vi "FRCts20_Backend_Test_Event_DELETE.vi"(8 "error in (no error)":errorcluster, 11 "Event Name":string) -> (0 "error out":errorcluster, 1 "Time (ms)":u32, 2 "Status":string, 3 "Event Out":T1, 5 "Success":bool)   [LabVIEW 2013, in "FRCts20_Backend_TestCode.lvlib"]
uses:
  FRCts20_Backend_TestCode.lvlib
  FRCts20_Backend_API/FRCts20_Backend_API_Event.ctl
  FRCts20_Backend_API/FRCts20_Backend_API_SW.ctl
  FRCts20_Backend_API/FRCts20_Backend_API_Command_Event.ctl
  FRCts20_Backend_API/FRCts20_Backend_API_Event.vi
  FRCts20_Backend_API/FRCts20_Backend_API.lvlib
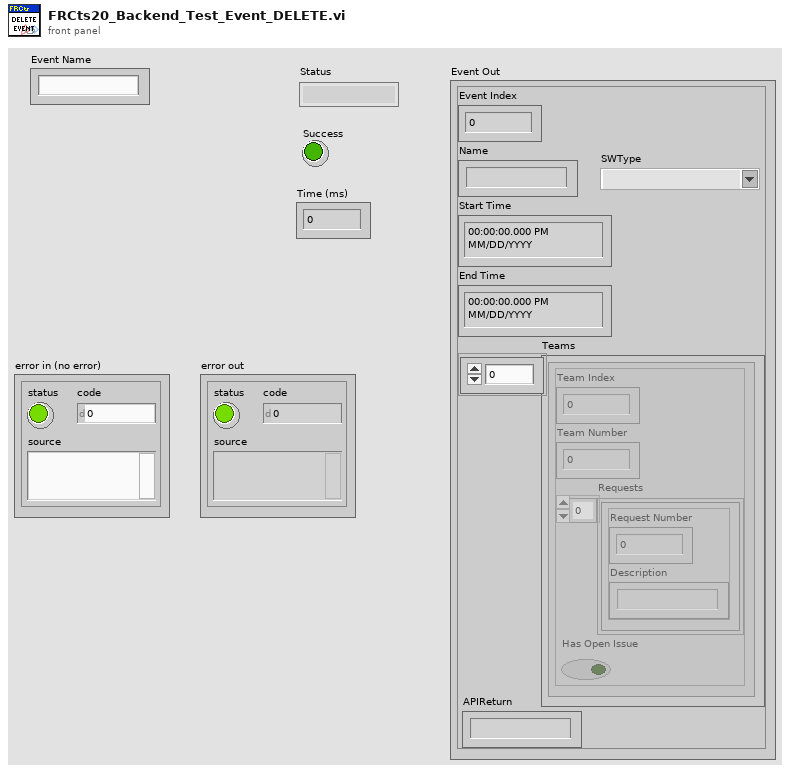
[diagram p1: front panel]
types:
  T1 = typedef "FRCts20_Backend_API.lvlib/FRCts20_Backend_API_Event.ctl" = cluster{"Event Index":u32, "Name":string, "Start Time":timestamp, "End Time":timestamp, "Teams":cluster{"Team Index":u32, "Team Number":u32, "Requests":cluster{"Request Number":u32, "Description":string}[], "Has Open Issue":bool}[], "SWType":T2, "APIReturn":string}
  T2 = typedef "FRCts20_Backend_API.lvlib/FRCts20_Backend_API_SW.ctl" = string
  T3 = typedef "FRCts20_Backend_API.lvlib/FRCts20_Backend_API_Command_Event.ctl" = string
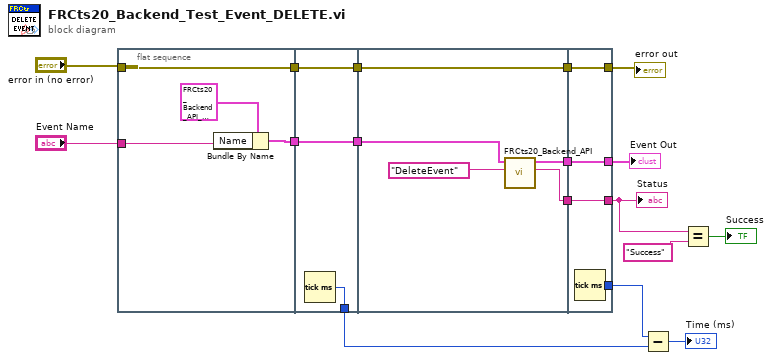
[diagram p0: block diagram]
diagram:
  n1 = flat-sequence {
    tunnel: "error in (no error)" -> [w21]
    tunnel: [w21] -> w17
    tunnel: [w20] -> w16
    tunnel: "Event Name" -> [w18]
    tunnel: [w24] -> w4
    tunnel: [w23] -> w15
    tunnel: w17 -> [w23]
    tunnel: [w22] -> w14
    tunnel: w16 -> [w22]
    tunnel: [w29] -> w13
    tunnel: w15 -> [w29]
    tunnel: w14 -> [w27]
    tunnel: [w26] -> w12
    tunnel: [w25] -> w11
    tunnel: [w33] -> w5
    tunnel: [w32] -> w7
    tunnel: w13 -> [w32]
    tunnel: [w31] -> w3
    tunnel: w12 -> [w31]
    tunnel: [w30] -> w2
    tunnel: w11 -> [w30]
    frame #0 {
      n2 = Bundle By Name(cluster=T1 {"Event Index"=0, "Name"="", "Start Time"=timestamp(0 s since 1904-01-01), "End Time"=timestamp(0 s since 1904-01-01), "Teams"=[], "SWType"="", "APIReturn"=""} ("Event In"), "Name"=w18) -> (w20:T1)
    }
    frame #1 {
      n3 = Tick Count (ms)() -> (millisecond timer value=w24:u32)
    }
    frame #2 {
      n4 = call-poly "FRCts20_Backend_API.vi"("Command"=T3 "DeleteEvent", "Event In"=w27) -> ("Status"=w25:string, "Event Out"=w26:T1)  [unwired: 7 in, 1 out]
    }
    frame #3 {
      n5 = Tick Count (ms)() -> (millisecond timer value=w33:u32)
    }
  }
  n6 = Subtract(x=w5, y=w4) -> (x-y=→"Time (ms)":u32)
  n7 = Equal?(x=w2, y="Success") -> (x = y?=→"Success":bool)
  "Event Out" <- w3
  "Status" <- w2
  "error out" <- w7
